vi "thcd_400_control.vi"() -> ()   [LabVIEW 2018]
uses:
  thcd_controls/ctrl_chn_thcd.ctl
  thcd_controls/ctrl_sms_thcd.ctl
  <vilib>/Utility/file.llb/Write Delimited Spreadsheet (DBL).vi
  thcd_commands/thcd_set_samp.vi
panel:
  out "thcd_st":bool
  out "thcd_res_msg":string
  in  "thcd_val":dbl min=0.0 max=100.0 step=1.0 format="%#.6g"
  out "ch3":dbl(graph)
  out "ch1":dbl(graph)
  out "ch2":dbl(graph)
  in  "milliseconds to wait":u32
  out "thcd_res_4":T2
  out "thcd_res_3":T2
  out "thcd_res_2":T2
  out "thcd_res_1":T2
  in  "getstat":bool
  in  "set":bool
  in  "read":bool
  out "res_val 3":dbl
  out "res_val 2":dbl
  out "res_val":dbl
  in  "Baud_rate":u32(ring)=19200 items=["9.6KHz"=9600, "19.2KHz"=19200]
  in  "thcd_visa":refnum<visa-resource-name>
  in  "Init Devices":bool
  in  "Exit":bool
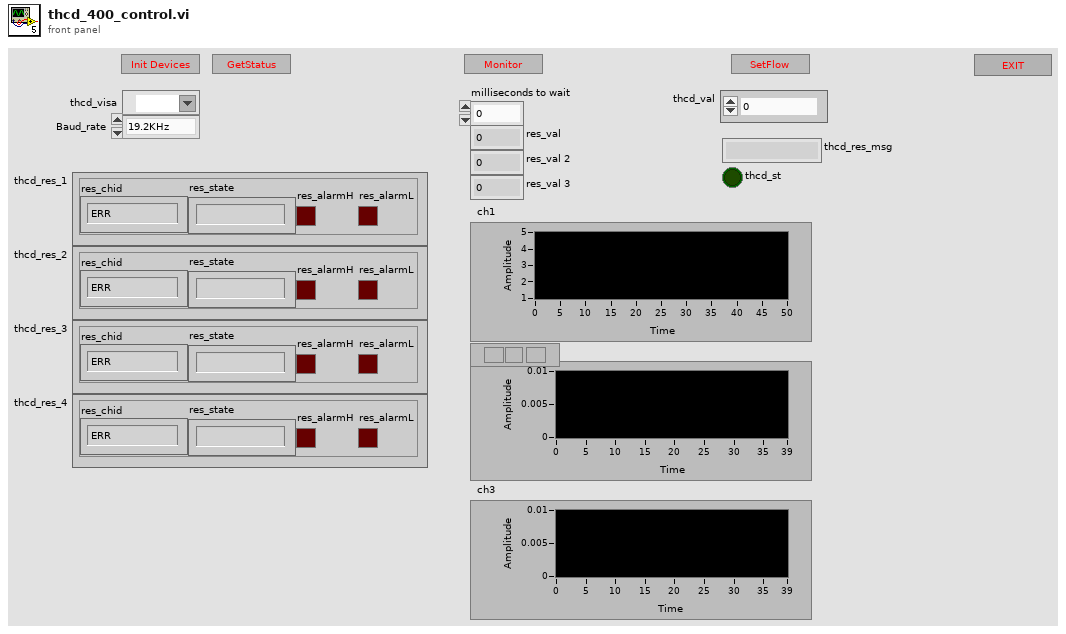
[diagram p1: front panel]
types:
  T1 = typedef "ctrl_chn_thcd.ctl" = enum8{"ERR", "1", "2", "3", "4"}
  T2 = cluster{"res_chid":T1, "res_state":string, "res_alarmH":bool, "res_alarmL":bool}
  T3 = typedef "ctrl_sms_thcd.ctl" = enum16{"idle", "init", "exit", "read", "set", "getstat"}
  T4 = enum16{"SetPoint", "AlarmH", "AlarmL", "Multiplier", "CalibValue"}
  T5 = cluster{"res_chid":T1, "res_val":dbl, "res_uom":string, "res_gid":string}[]
  T6 = cluster{"res_chid":T1, "res_val":dbl, "res_uom":string, "res_gid":string}
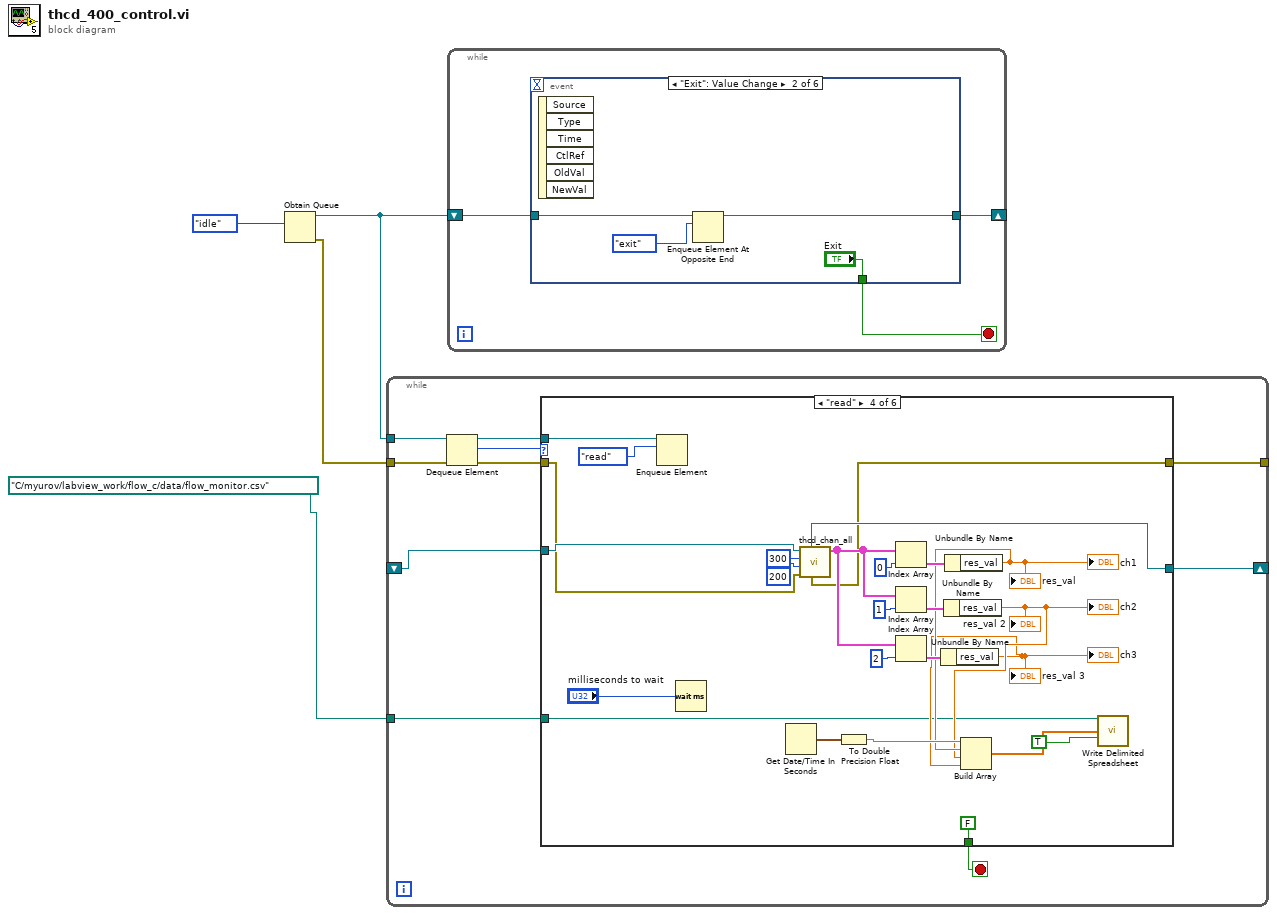
[diagram p0: block diagram]
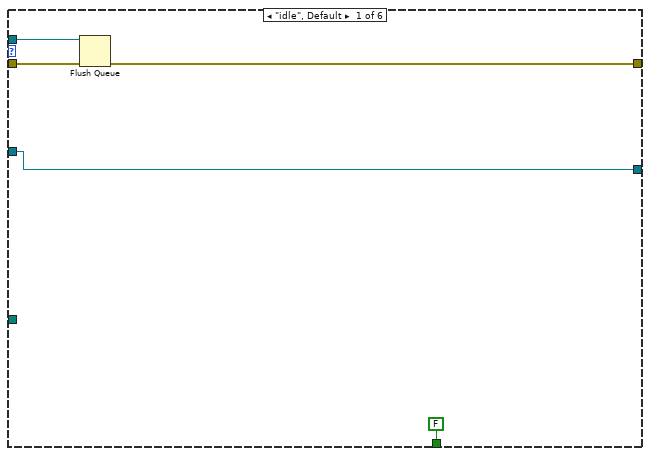
[diagram p2: hidden frame]
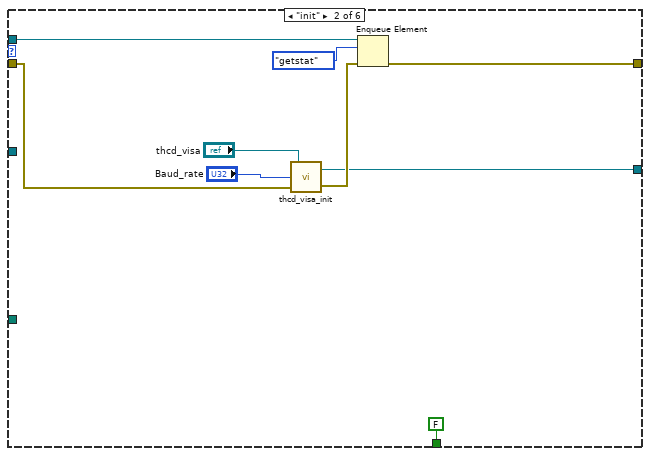
[diagram p3: hidden frame]
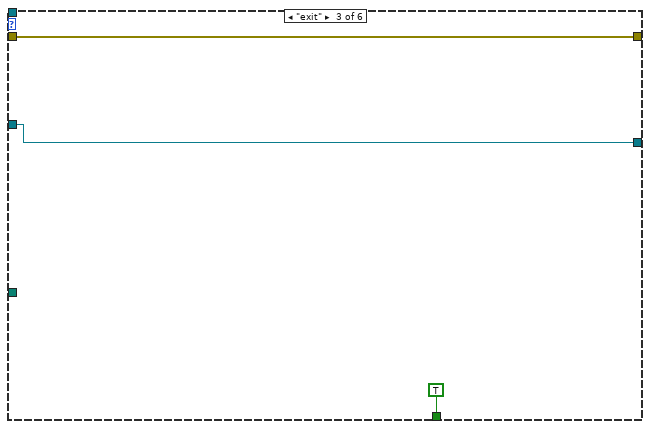
[diagram p4: hidden frame]
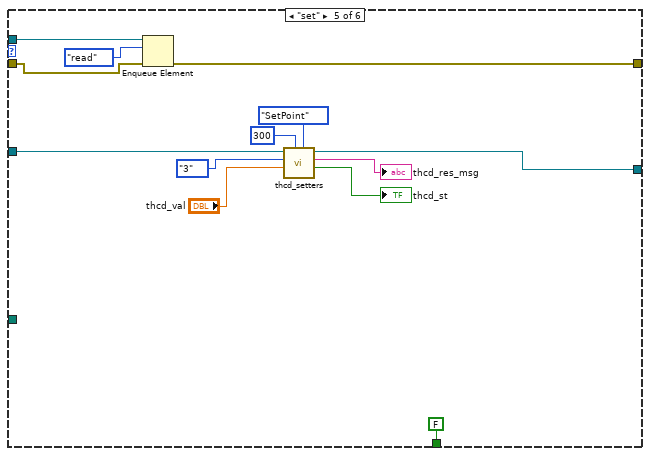
[diagram p5: hidden frame]
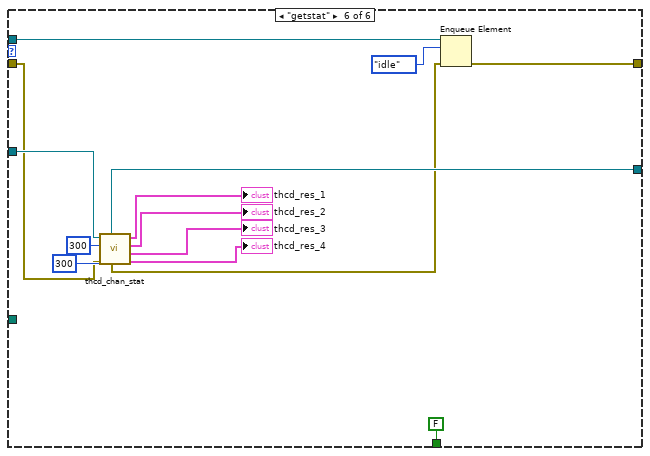
[diagram p6: hidden frame]
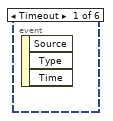
[diagram p7: hidden frame]
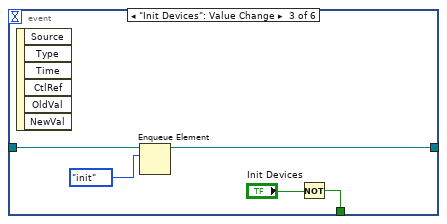
[diagram p8: hidden frame]
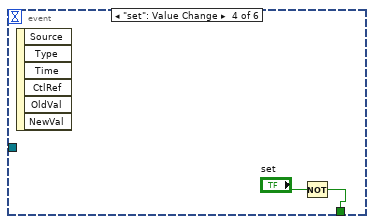
[diagram p9: hidden frame]
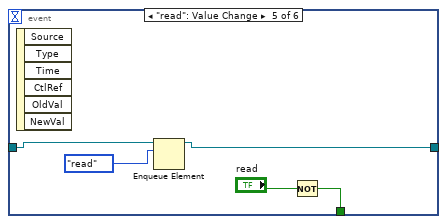
[diagram p10: hidden frame]
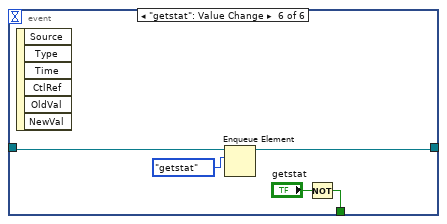
[diagram p11: hidden frame]
diagram:
  n1 = Obtain Queue(element data type=ctrl_sms_thcd."idle" ("Enum")) -> (queue out=w3:refnum<queue>, error out=w2:errorcluster)  [unwired: 4 in, 1 out]
  n2 = while {
    tunnel: w2 -> [w12]
    tunnel: [w9] -> _
    tunnel: w3 -> [w13]
    shift-right: [w7] -> _
    shift-left: _ -> [w6]
    tunnel: path "C:/myurov/labview_work/flow_c/data/flow_monitor.csv" ("file path (dialog if empty)") -> [w5]
    stop <- w14 stop-if-true
    n3 = Dequeue Element(queue=w13, error in (no error)=w12) -> (queue out=w8:refnum<queue>, element=w11:T3, error out=w10:errorcluster)  [unwired: 1 in, 1 out]
    n4 = case shown="\"read\"" w11 {
      tunnel: w8 -> [w18 w24 _ w40 w67 w73]
      tunnel: [FALSE FALSE TRUE FALSE FALSE FALSE] -> w14
      tunnel: w10 -> [w17 w25 w30 w55 w66 w79]
      tunnel: [w16 w21 w30 w44 w65 w71] -> w9
      tunnel: [w15 w20 w29 w52 w63 w82] -> w7
      tunnel: w6 -> [w15 _ w29 w56 w64 w83]
      tunnel: w5 -> [_ _ _ w32 _ _]
      frame "idle", Default {
        n5 = Flush Queue(queue=w18, error in (no error)=w17) -> (error out=w16:errorcluster)  [unwired: 2 out]
      }
      frame "init" {
        n6 = call "thcd_visa_init.vi"("err_in"=w25, "Serial Settings:Baud Rate"="Baud_rate", "thcd_visa"="thcd_visa") -> ("err_out"=w22:errorcluster, "thcd_visa"=w20:refnum<visa-resource-name>)
        n7 = Enqueue Element(queue=w24, element=ctrl_sms_thcd."getstat", error in (no error)=w22) -> (error out=w21:errorcluster)  [unwired: 1 in, 2 out]
      }
      frame "exit" {
      }
      frame "read" {
        n8 = Enqueue Element(queue=w40, element=ctrl_sms_thcd."read") -> ()  [unwired: 2 in, 3 out]
        n9 = Wait (ms)(milliseconds to wait="milliseconds to wait") -> ()  [unwired: 1 out]
        n10 = Get Date/Time In Seconds() -> (seconds since 1Jan1904=w39:timestamp)
        n11 = call "thcd_chan_all.vi"("err_in"=w55, "thcd_b2r"=u32 200, "thcd_delay"=u32 300, "thcd_visa"=w56) -> ("thcd_res"=w45:T5, "err_out"=w44:errorcluster, "thcd_visa"=w52:refnum<visa-resource-name>)  [unwired: 3 in, 2 out]
        n12 = To Double Precision Float(number=w39) -> (double precision float=w36:dbl)
        n13 = Index Array(array=w45, index=0) -> (element=w50:T6)
        n14 = Index Array(array=w45, index=1) -> (element=w49:T6)
        n15 = Index Array(array=w45, index=2) -> (element=w48:T6)
        n16 = Unbundle By Name(w48) -> ("res_val"=w33:dbl)
        "res_val 3" <- w33
        "ch3" <- w33
        n17 = Unbundle By Name(w49) -> ("res_val"=w34:dbl)
        "res_val 2" <- w34
        "ch2" <- w34
        n18 = Unbundle By Name(w50) -> ("res_val"=w35:dbl)
        "res_val" <- w35
        "ch1" <- w35
        n19 = Build Array(w36, w35, w34, w33) -> (w38:dbl[])
        n20 = call-poly <vilib>:"Write Delimited Spreadsheet.vi"("file path (dialog if empty)"=w32, "1D data"=w38, "append to file? (new file:F)"=TRUE ("append to file? (F)")) -> ()  [unwired: 11 in, 2 out]
      }
      frame "set" {
        n21 = Enqueue Element(queue=w67, element=ctrl_sms_thcd."read", error in (no error)=w66) -> (error out=w65:errorcluster)  [unwired: 1 in, 2 out]
        n22 = call-poly "thcd_setters.vi"("thcd_com"=T4."SetPoint", "thcd_delay"=u32 300, "thcd_val"="thcd_val", "thcd_ch"=ctrl_chn_thcd."3", "thcd_visa"=w64) -> ("thcd_st"=→"thcd_st":bool, "thcd_res_msg"=→"thcd_res_msg":string, "thcd_visa"=w63:refnum<visa-resource-name>)  [unwired: 1 in, 1 out]
      }
      frame "getstat" {
        n23 = call "thcd_chan_stat.vi"("err_in"=w79, "thcd_b2r"=u32 300, "thcd_delay"=u32 300, "thcd_visa"=w83) -> ("thcd_res_4"=→"thcd_res_4":T2, "thcd_res_3"=→"thcd_res_3":T2, "thcd_res_2"=→"thcd_res_2":T2, "thcd_res_1"=→"thcd_res_1":T2, "err_out"=w72:errorcluster, "thcd_visa"=w82:refnum<visa-resource-name>)  [unwired: 2 out]
        n24 = Enqueue Element(queue=w73, element=ctrl_sms_thcd."idle", error in (no error)=w72) -> (error out=w71:errorcluster)  [unwired: 1 in, 2 out]
      }
    }
  }
  n25 = while {
    shift-right: [w85] -> _
    shift-left: w3 -> [w86]
    stop <- w84 stop-if-true
    n26 = event shown="[1] \"Exit\": Value Change" {
      selector: _ -> [_ _ _ _ _ _]
      dyn-events: _ -> [_ _ _ _ _ _]
      timeout: _ -> [_ _ _ _ _ _]
      tunnel: w86 -> [_ w90 w95 _ w100 w105]
      tunnel: [_ w89 w94 _ w99 w104] -> w85
      tunnel: [_ "Exit" w91 w96 w101 w106] -> w84
      event Timeout {
        n27 = event-data() -> ()  [unwired: 1 in, 3 out]
      }
      event "Exit": Value Change {
        n28 = event-data() -> ()  [unwired: 1 in, 6 out]
        n29 = Enqueue Element At Opposite End(queue=w90, element=ctrl_sms_thcd."exit" ("Enum")) -> (queue out=w89:refnum<queue>)  [unwired: 2 in, 2 out]
      }
      event "Init Devices": Value Change {
        n30 = event-data() -> ()  [unwired: 1 in, 6 out]
        n31 = Enqueue Element(queue=w95, element=ctrl_sms_thcd."init") -> (queue out=w94:refnum<queue>)  [unwired: 2 in, 2 out]
        n32 = Not(x="Init Devices") -> (.not. x?=w91:bool)
      }
      event "set": Value Change {
        n33 = event-data() -> ()  [unwired: 1 in, 6 out]
        n34 = Not(x="set") -> (.not. x?=w96:bool)
      }
      event "read": Value Change {
        n35 = event-data() -> ()  [unwired: 1 in, 6 out]
        n36 = Enqueue Element(queue=w100, element=ctrl_sms_thcd."read" ("Enum")) -> (queue out=w99:refnum<queue>)  [unwired: 2 in, 2 out]
        n37 = Not(x="read") -> (.not. x?=w101:bool)
      }
      event "getstat": Value Change {
        n38 = event-data() -> ()  [unwired: 1 in, 6 out]
        n39 = Enqueue Element(queue=w105, element=ctrl_sms_thcd."getstat") -> (queue out=w104:refnum<queue>)  [unwired: 2 in, 2 out]
        n40 = Not(x="getstat") -> (.not. x?=w106:bool)
      }
    }
  }
